vi "ComputeWfmScalar.vi"(6 "GrpCfg":T1, 7 "Speed":T2, 8 "error in (no error)":errorcluster, 10 "Y Array":sgl[](array[numeric]), 11 "Tachometer in":refnum<class "Tachometer.lvclass">) -> (0 "error out":errorcluster, 2 "Metric":dbl, 3 "Tachometer Out":refnum<class "Tachometer.lvclass">)   [LabVIEW 2018, in "Measurement Channels.lvlib" / "Tachometer.lvclass"]
uses:
  Tachometer.lvclass
  C:/Users/Jeff Tipps/Documents/DAQMan/source/Classes/Measurements/Class Frequency/Frequency.lvclass
  Common/Controls/TE_Designator.ctl
  Common/Controls/Group Timing Info.ctl
  Tachometer.lvclass/Tachometer.ctl
  Class Frequency/Read Min EU.vi
  Class Frequency/Read Slope.vi
  Class Frequency/Read Thresh.vi
  Class Frequency/Read AnalogTach States.vi
  Class Frequency/Read Speed From Pulse State.vi
  Class Frequency/Write AnalogTach States.vi
  Class Frequency/Write Speed From Pulse State.vi
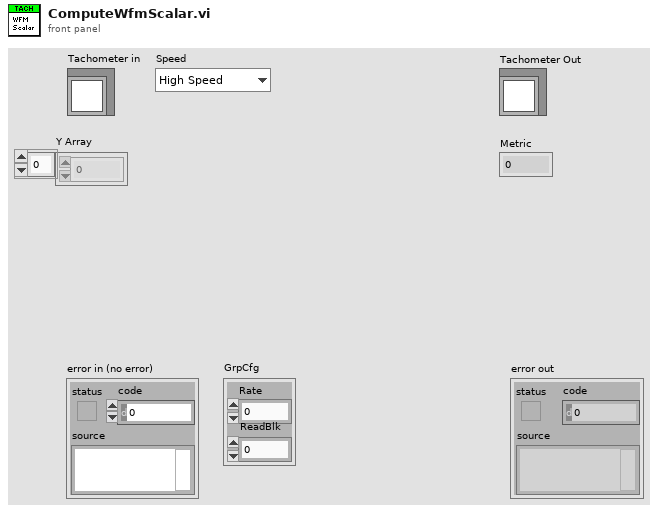
[diagram p1: front panel]
types:
  T1 = typedef "Group Timing Info.ctl" = cluster{"Rate":dbl, "ReadBlk":i32}
  T2 = typedef "TE_Designator.ctl" = enum16{"High Speed", "Low Speed"}
  T3 = cluster{"Analog Tach State":dbl, "Edge Detection State":cluster{"processed data":dbl, "buffer data":dbl[]}, "Reset?":bool}
  T4 = cluster{"state":enum16{"0 Pulses", "1 Pulse", "2+ Pulses"}, "last pulse position":dbl, "RPM":dbl, "Empty Blocks":i32}
  T5 = typedef "OAT Position Info.ctl" = cluster{"positions [s]":dbl[], "samples/rev":dbl}
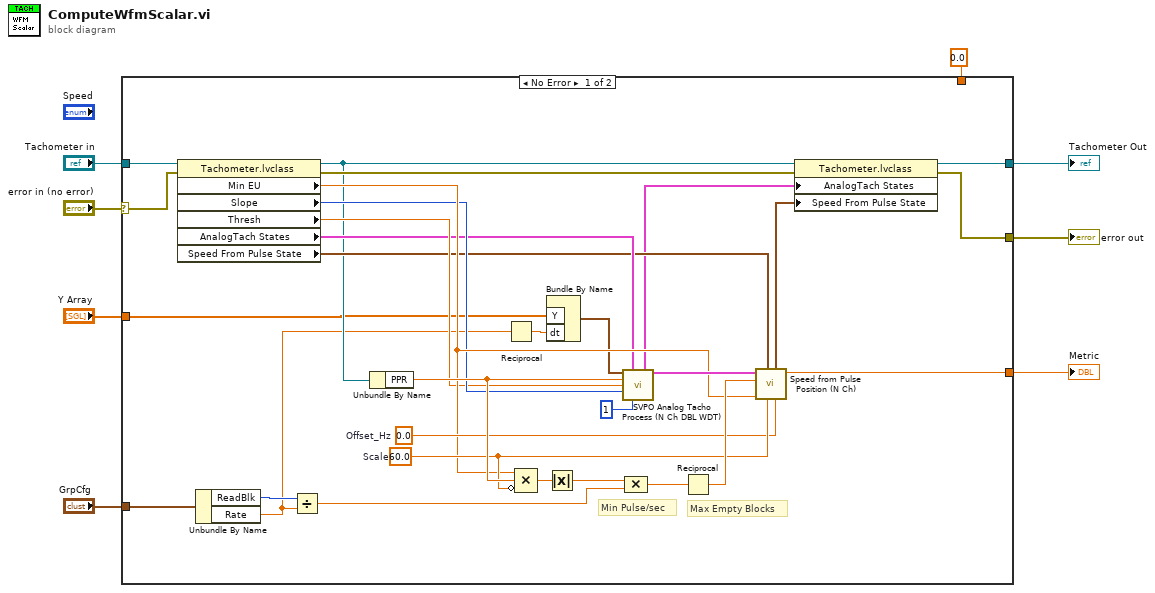
[diagram p0: block diagram]
diagram:
  n1 = case shown="No Error" "error in (no error)" {
    selector: "error in (no error)" -> [w26 w41]
    tunnel: [w30 w40] -> w8
    tunnel: "GrpCfg" -> [w16 _]
    tunnel: "Y Array" -> [w13 _]
    tunnel: "Tachometer in" -> [w19 w39]
    tunnel: [w17 w41] -> w4
    tunnel: 0.0 ("Speed in EU") -> [_ w40]
    tunnel: [w18 w39] -> w1
    frame No Error {
      w33 = 0.0  # Offset_Hz
      w34 = 60.0  # Scale
      # "Max Empty Blocks"
      # "Min Pulse/sec"
      n2 = property class="Tachometer.lvclass"(reference=w19, error in=w26) -> (reference out=w22:refnum<class "Tachometer.lvclass">, error out=w23:errorcluster, "Min EU"=w29:dbl, "Slope"=w28:u16, "Thresh"=w27:dbl, "AnalogTach States"=w25:T3, "Speed From Pulse State"=w24:T4)
      n3 = Unbundle By Name(w16) -> ("ReadBlk"=w15:i32, "Rate"=w10:dbl)
      n4 = Divide(x=w15, y=w10) -> (x/y=w14:dbl)
      n5 = Unbundle By Name(w22) -> ("PPR"=w37:dbl)
      n6 = Reciprocal(x=w10) -> (1/x=w11:dbl)
      n7 = Compound Arithmetic op=MULTIPLY(w29, w37, invert w34) -> (w32:dbl)
      n8 = Bundle By Name("Y"=w13, "dt"=w11) -> (w12:waveform(sgl))  [unwired: 1 in]
      n9 = Absolute Value(x=w32) -> (abs(x)=w31:dbl)
      n10 = call "SVPO Analog Tacho Process (N Ch DBL WDT).vi"("analog tacho signal"=w12, "AnalogTach States"=w25, "PPR"=w37, "Thresh(V)"=w27, "Slope"=w28, "pulse width (2)"=1) -> ("AnalogTach States Out"=w21:T3, "speed position info"=w38:T5)  [unwired: 8 in]
      n11 = Compound Arithmetic op=MULTIPLY(w31, w14) -> (w36:dbl)
      n12 = Reciprocal(x=w36) -> (1/x=w35:dbl)
      n13 = call "Speed from Pulse Position (N Ch).vi"("Offset"=w33, "Scale"=w34, "Speed From Pulse"=w24, "Min EU"=w29, "Max Empty Blocks"=w35, "speed position info"=w38) -> ("Speed in EU"=w30:dbl, "Speed From Pulse"=w20:T4)  [unwired: 4 in]
      n14 = property class="Tachometer.lvclass"(reference=w22, error in=w23, "AnalogTach States"=w21, "Speed From Pulse State"=w20) -> (reference out=w18:refnum<class "Tachometer.lvclass">, error out=w17:errorcluster)
    }
    frame Error {
    }
  }
  "error out" <- w4
  "Metric" <- w8
  "Tachometer Out" <- w1
